vi "Stop Core.vi"(10 "final error code":i32, 11 "Cooler in":refnum<class "Cooler.lvclass">) -> (3 "Cooler out":refnum<class "Cooler.lvclass">)   [LabVIEW 2012, in "Cooler.lvlib" / "Cooler.lvclass"]
doc: "In override VIs of Stop Core.vi, an actor should invoke any code needed to stop all the parallel processes that it created during its run. This includes any nested actors that it created and any other asynchronously running VIs, such as a Time-Delated Message. It may also include all parallel loops in its Actor Core, although it is acceptable to stop those using a local signal on the Actor Core block diagram that is raised after the Call Parent Node finishes. \n\nThe <b>final error code</b> input tells the actor what error was set when this actor quit. Zero means there was no error. You can use this to decide whether this should be treated as a Normal Stop or an Emergency Stop for the purposes of signaling other actors. In general, any non-zero value should be treated as an Emergency Stop, though a given actor is free to choose other policies. Note that the particular error code 1608 indicates that this actor was itself stopped by an Emergency Stop and should pass that along."
uses:
  Cooler.lvclass
  Level Controller/Level Controller/Level Controller.lvclass
  Cooler.lvclass/Cooler.ctl
  <vilib>/ActorFramework/Stop Msg/Stop Msg.lvclass/Stop Msg.ctl
  <vilib>/ActorFramework/Message Enqueuer/Message Enqueuer.lvclass/Message Enqueuer.ctl
  <vilib>/ActorFramework/Stop Msg/Send Emergency Stop.vi
  <vilib>/ActorFramework/Stop Msg/Send Normal Stop.vi
  <vilib>/ActorFramework/Message Enqueuer/Enqueue Critical.vi
  <vilib>/ActorFramework/Message Enqueuer/Enqueue.vi
  <vilib>/ActorFramework/Message Priority Queue/Priority Enqueue.vi
  <vilib>/ActorFramework/Stop Msg/Stop Msg.lvclass
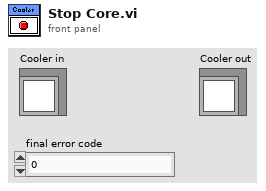
[diagram p1: front panel]
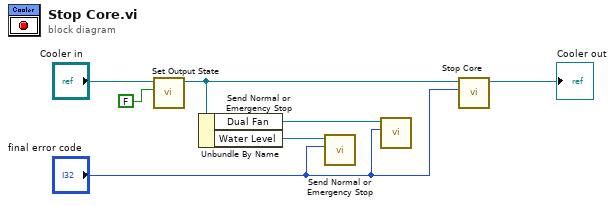
[diagram p0: block diagram]
diagram:
  n1 = call-dynamic "Set Output State.vi"("Output State"=FALSE, "Cooler in"="Cooler in") -> ("Cooler out"=w6:refnum<class "Cooler.lvclass">)  [unwired: 8 in, 1 out]
  n2 = Unbundle By Name(w6) -> ("Dual Fan"=w3:refnum<class "Message Enqueuer.lvclass">, "Water Level"=w2:refnum<class "Message Enqueuer.lvclass">)
  n3 = call <vilib>:"Send Normal or Emergency Stop.vi"("final error code"="final error code", "Message Enqueuer"=w2) -> ()  [unwired: 9 in, 1 out]
  n4 = call <vilib>:"Send Normal or Emergency Stop.vi"("final error code"="final error code", "Message Enqueuer"=w3) -> ()  [unwired: 9 in, 1 out]
  n5 = call-parent "Stop Core.vi"("final error code"="final error code", "Actor in"=w6) -> ("Actor out"=→"Cooler out":refnum<class "Cooler.lvclass">)  [unwired: 9 in]
